vi "Init_Params.vi"(0 "dimension":i32=3, 2 "#hidden_units":i32=2, 5 "Scale Factor":dbl=1.0 format="%_8f") -> (16 "h_init":T1, 18 "params":T2={"Wxh"=[[0.24470252823431293, 0.04918857305855216, 0.48683434931773895], [-0.9102380385787178, -1.367873529790151, -0.20526552882366572]], "Whh"=[[0.49264123363313495, 0.5132642197032382], [0.7043975290480302, -0.8166023631999548]], "bh"=[[-0.05214115137580276], [0.7025112491086567]], "Why"=[[0.9124809061676967, -1.7618279045577308], [-0.4746242092582831, 0.7935987850266535], [-0.425664601601623, -0.5320526538057628]], "by"=[[-1.2247915013883226], [0.48850202961995576], [-0.7909583487350551]]} {"Wxh" format="%_8f"; "Whh" format="%_8f"; "bh" format="%_8f"; "Why" format="%_8f"; "by" format="%_8f"})   [LabVIEW 2014]
uses:
  <vilib>/Analysis/Matrix/Datatypes/RealMatrix.ctl
  <vilib>/Analysis/Matrix/NI_Matrix.lvlib
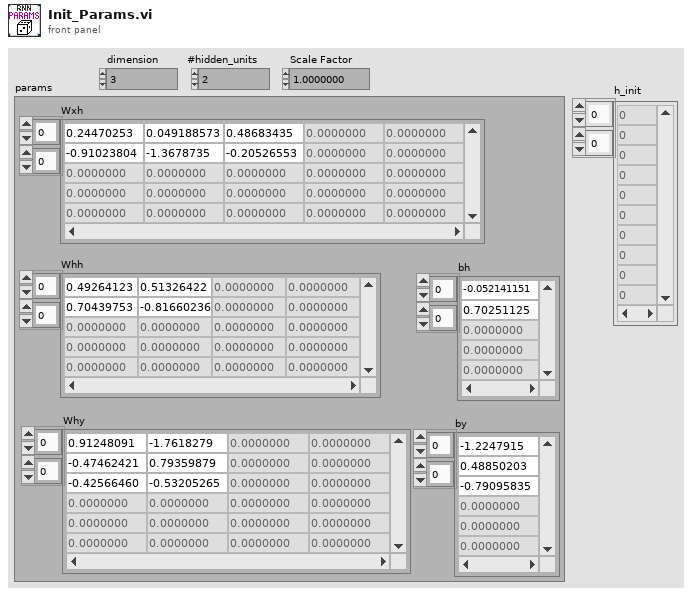
[diagram p1: front panel]
types:
  T1 = typedef "NI_Matrix.lvlib/RealMatrix.ctl" = dbl[][]
  T2 = cluster{"Wxh":T1, "Whh":T1, "bh":T1, "Why":T1, "by":T1}
  T3 = cluster{"Scaled Matrix":T1, "Scaled Matrix":T1, "Scaled Matrix":T1, "Scaled Matrix":T1, "Scaled Matrix":T1}
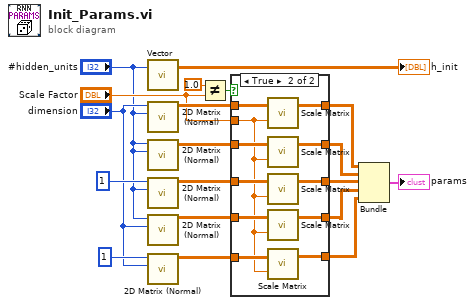
[diagram p0: block diagram]
diagram:
  n1 = call "Vector.vi"("length"="#hidden_units") -> ("Real Matrix (Column Vector)"=→"h_init":T1)  [unwired: 18 in]
  n2 = call "2D Matrix (Normal).vi"("nRows"="#hidden_units", "nCols"="dimension") -> ("Normal Matrix"=w15:T1)  [unwired: 9 in]
  n3 = call "2D Matrix (Normal).vi"("nRows"="#hidden_units", "nCols"="#hidden_units") -> ("Normal Matrix"=w13:T1)  [unwired: 9 in]
  n4 = call "2D Matrix (Normal).vi"("nRows"="#hidden_units", "nCols"=1) -> ("Normal Matrix"=w12:T1)  [unwired: 9 in]
  n5 = call "2D Matrix (Normal).vi"("nRows"="dimension", "nCols"="#hidden_units") -> ("Normal Matrix"=w11:T1)  [unwired: 9 in]
  n6 = call "2D Matrix (Normal).vi"("nRows"="dimension", "nCols"=1) -> ("Normal Matrix"=w10:T1)  [unwired: 9 in]
  n7 = Not Equal?(x=1.0, y="Scale Factor") -> (x != y?=w5:bool)
  n8 = case shown="True" w5 {
    tunnel: w15 -> [w24 w35]
    tunnel: [w24 w34] -> w14
    tunnel: w13 -> [w23 w33]
    tunnel: w12 -> [w22 w32]
    tunnel: w11 -> [w21 w31]
    tunnel: w10 -> [w20 w30]
    tunnel: "Scale Factor" -> [_ w29]
    tunnel: [w23 w28] -> w9
    tunnel: [w22 w27] -> w8
    tunnel: [w21 w26] -> w7
    tunnel: [w20 w25] -> w6
    frame False {
    }
    frame True {
      n9 = call "Scale Matrix.vi"("Matrix"=w35, "Scale Factor"=w29) -> ("Scaled Matrix"=w34:T1)  [unwired: 17 in]
      n10 = call "Scale Matrix.vi"("Matrix"=w33, "Scale Factor"=w29) -> ("Scaled Matrix"=w28:T1)  [unwired: 17 in]
      n11 = call "Scale Matrix.vi"("Matrix"=w32, "Scale Factor"=w29) -> ("Scaled Matrix"=w27:T1)  [unwired: 17 in]
      n12 = call "Scale Matrix.vi"("Matrix"=w31, "Scale Factor"=w29) -> ("Scaled Matrix"=w26:T1)  [unwired: 17 in]
      n13 = call "Scale Matrix.vi"("Matrix"=w30, "Scale Factor"=w29) -> ("Scaled Matrix"=w25:T1)  [unwired: 17 in]
    }
  }
  n14 = Bundle("Scaled Matrix"=w14, "Scaled Matrix"=w9, "Scaled Matrix"=w8, "Scaled Matrix"=w7, "Scaled Matrix"=w6) -> (→"params":T3)  [unwired: 1 in]
